vi "Decodifica_Msg.vi"(1 "Msg":string) -> (3 "Volts":dbl, 4 "Graus":dbl, 5 "Intensitat":dbl)   [LabVIEW 2017]
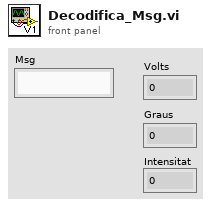
[diagram p1: front panel]
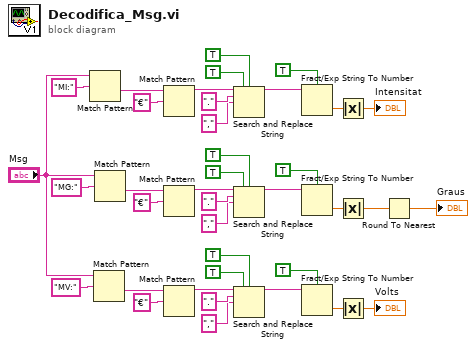
[diagram p0: block diagram]
diagram:
  n1 = Match Pattern(string="Msg", regular expression="MI:") -> (after substring=w21:string)  [unwired: 1 in, 3 out]
  n2 = Match Pattern(string="Msg", regular expression="MV:") -> (after substring=w38:string)  [unwired: 1 in, 3 out]
  n3 = Match Pattern(string="Msg", regular expression="MG:") -> (after substring=w30:string)  [unwired: 1 in, 3 out]
  n4 = Match Pattern(string=w21, regular expression="€") -> (before substring=w17:string)  [unwired: 1 in, 3 out]
  n5 = Match Pattern(string=w30, regular expression="€") -> (before substring=w26:string)  [unwired: 1 in, 3 out]
  n6 = Match Pattern(string=w38, regular expression="€") -> (before substring=w35:string)  [unwired: 1 in, 3 out]
  n7 = Search and Replace String(replace all?=TRUE ("replace all? (F)"), case sensitive?=TRUE ("ignore case? (F)"), input string=w17, search string=".", replace string="," ("replace string (\"\")")) -> (result string=w1:string)  [unwired: 3 in, 3 out]
  n8 = Search and Replace String(replace all?=TRUE ("replace all? (F)"), case sensitive?=TRUE ("ignore case? (F)"), input string=w26, search string=".", replace string="," ("replace string (\"\")")) -> (result string=w3:string)  [unwired: 3 in, 3 out]
  n9 = Search and Replace String(replace all?=TRUE ("replace all? (F)"), case sensitive?=TRUE ("ignore case? (F)"), input string=w35, search string=".", replace string="," ("replace string (\"\")")) -> (result string=w2:string)  [unwired: 3 in, 3 out]
  n10 = Fract/Exp String To Number(use system decimal point (T)=TRUE, string=w1) -> (number=w12:dbl)  [unwired: 2 in, 1 out]
  n11 = Fract/Exp String To Number(use system decimal point (T)=TRUE, string=w3) -> (number=w8:dbl)  [unwired: 2 in, 1 out]
  n12 = Fract/Exp String To Number(use system decimal point (T)=TRUE, string=w2) -> (number=w10:dbl)  [unwired: 2 in, 1 out]
  n13 = Absolute Value(x=w12) -> (abs(x)=→"Intensitat":dbl)
  n14 = Absolute Value(x=w8) -> (abs(x)=w6:dbl)
  n15 = Absolute Value(x=w10) -> (abs(x)=→"Volts":dbl)
  n16 = Round To Nearest(number=w6) -> (nearest integer value=→"Graus":dbl)
